vi "Get CAN Interface Status.vi"(8 "error in":errorcluster, 11 "HSU MCU V2 Monitor CFG in":refnum<class "HSU MCU V2 CFG.lvclass">) -> (0 "error out":errorcluster, 2 "function return":u32, 3 "HSU MCU V2 Monitor CFG out":refnum<class "HSU MCU V2 CFG.lvclass">)   [LabVIEW 2023, in "HSU MCU V2 CFG.lvclass"]
uses:
  HSU MCU V2 CFG.lvclass
  HSU MCU V2 CFG.lvclass/HSU MCU V2 CFG.ctl
  CAN Interfaces/PCAN/PCAN.lvclass
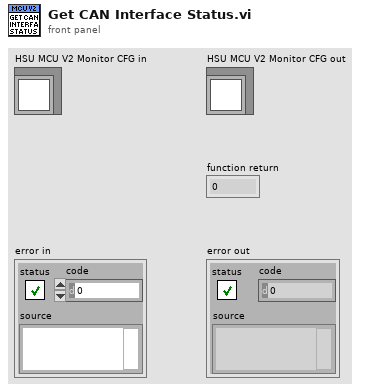
[diagram p1: front panel]
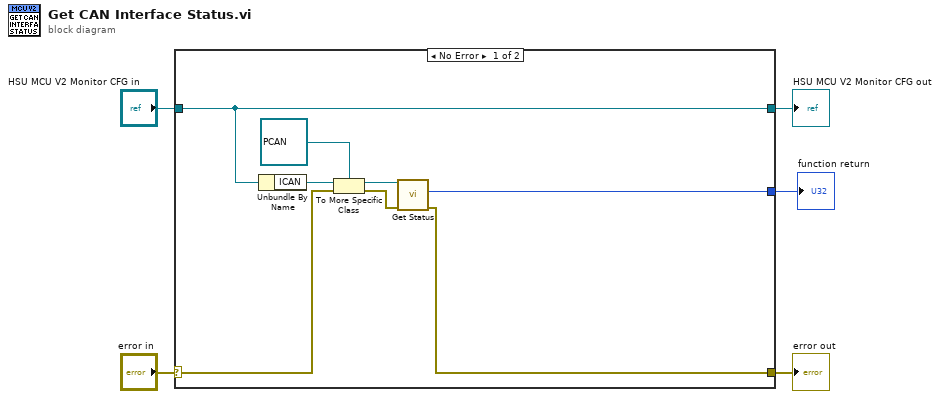
[diagram p0: block diagram]
diagram:
  n1 = case shown="No Error" "error in" {
    selector: "error in" -> [w7 w15]
    tunnel: [w6 w15] -> w4
    tunnel: [w13 w14] -> w2
    tunnel: "HSU MCU V2 Monitor CFG in" -> [w13 w14]
    tunnel: [w8 _] -> w1
    frame No Error {
      n2 = Unbundle By Name(w13) -> ("ICAN"=w12:refnum<class "ICAN.lvclass">)
      n3 = To More Specific Class(target class=refnum<class "PCAN.lvclass"> refnum ("PCAN.lvclass"), reference=w12, error in=w7) -> (specific class reference=w10:refnum<class "PCAN.lvclass">, error out=w9:errorcluster)
      n4 = call "Get Status.vi"("error in"=w9, "PCAN in"=w10) -> ("error out"=w6:errorcluster, "function return"=w8:u32)  [unwired: 7 in, 1 out]
    }
    frame Error {
    }
  }
  "error out" <- w4
  "HSU MCU V2 Monitor CFG out" <- w2
  "function return" <- w1
